vi "Create GCF LUT.vi"(8 "error in (no error)":errorcluster, 11 "C100L in":refnum<class "C100L.lvclass">) -> (0 "error out":errorcluster, 3 "C100L out":refnum<class "C100L.lvclass">)   [LabVIEW 2021, in "C100L.lvlib" / "C100L.lvclass"]
uses:
  C100L.lvclass
  GCF Data.ctl
  C100L.lvclass/C100L.ctl
  <vilib>/Utility/file.llb/Read Delimited Spreadsheet (string).vi
  <vilib>/BenjaminR/LookUp Table API/LUT.lvclass
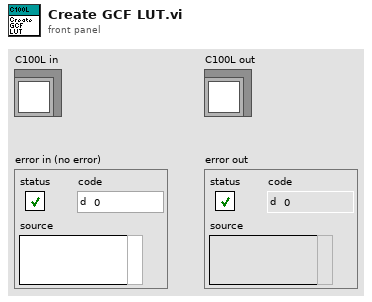
[diagram p1: front panel]
types:
  T1 = typedef "C100L.lvlib/C100L.lvclass/GCF Data.ctl" = map{string, dbl}
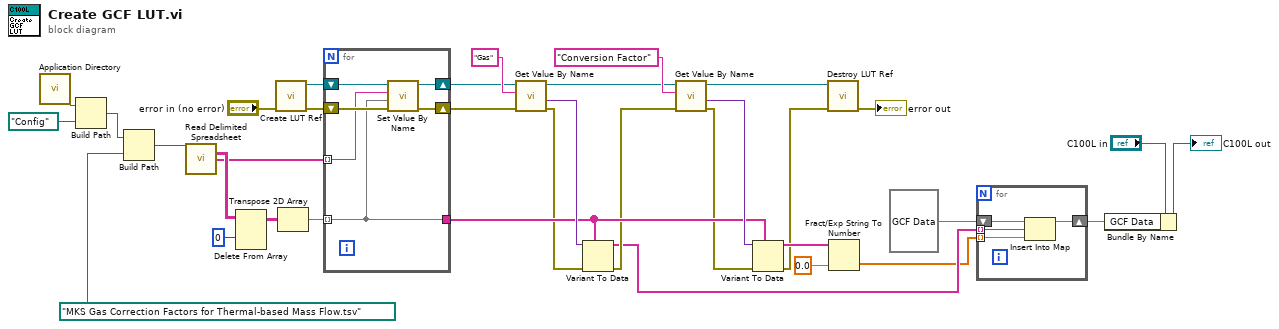
[diagram p0: block diagram]
diagram:
  n1 = call <vilib>:"Application Directory.vi"() -> ("Application Directory"=w5:path)
  n2 = Build Path(base path=w5, name or relative path=path "Config") -> (appended path=w3:path)
  n3 = Build Path(base path=w3, name or relative path=path "MKS Gas Correction Factors for Thermal-based Mass Flow.tsv" ("file path (dialog if empty)")) -> (appended path=w1:path)
  n4 = call-poly <vilib>:"Read Delimited Spreadsheet.vi"("file path (dialog if empty)"=w1) -> ("all rows"=w35:string[][], "first row"=w32:string[])  [unwired: 9 in, 4 out]
  n5 = Delete From Array(array=w35, index (row)=0) -> (array with subset deleted=w30:string[][])  [unwired: 2 in, 1 out]
  n6 = call <vilib>:"Create LUT Ref.vi"("error in (no error)"="error in (no error)") -> ("error out"=w31:errorcluster, "LUT out"=w33:refnum<class "LUT.lvclass">)  [unwired: 9 in]
  n7 = Transpose 2D Array(2D array=w30) -> (transposed array=w29:string[][])
  n8 = for {
    tunnel: w32 -> [w37] mode=indexing
    tunnel: w29 -> [w36] mode=indexing
    shift-right: [w40] -> w26
    shift-left: w33 -> [w41]
    shift-right: [w39] -> w27
    shift-left: w31 -> [w38]
    tunnel: [w36] -> w21
    n9 = call <vilib>:"Set Value By Name.vi"("error in (no error)"=w38, "Value"=w36, "Name"=w37, "LUT in"=w41) -> ("error out"=w39:errorcluster, "LUT out"=w40:refnum<class "LUT.lvclass">)  [unwired: 5 in, 1 out]
  }
  n10 = call <vilib>:"Get Value By Name.vi"("error in (no error)"=w27, "Name"="Gas", "LUT in"=w26) -> ("error out"=w15:errorcluster, "Value"=w25:variant, "LUT out"=w22:refnum<class "LUT.lvclass">)  [unwired: 5 in, 1 out]
  n11 = Variant To Data(error in=w15, type=w21, Variant=w25) -> (data=w9:string[], error out=w14:errorcluster)
  n12 = call <vilib>:"Get Value By Name.vi"("error in (no error)"=w14, "Name"="Conversion Factor", "LUT in"=w22) -> ("error out"=w13:errorcluster, "Value"=w24:variant, "LUT out"=w18:refnum<class "LUT.lvclass">)  [unwired: 5 in, 1 out]
  n13 = Variant To Data(error in=w13, type=w21, Variant=w24) -> (data=w20:string[], error out=w12:errorcluster)
  n14 = call <vilib>:"Destroy LUT Ref.vi"("error in (no error)"=w12, "LUT in"=w18) -> ("error out"=→"error out":errorcluster)  [unwired: 9 in]
  n15 = Fract/Exp String To Number(string=w20, default (0 dbl)=0.0 ("default (0 DBL)")) -> (number=w8:dbl[])  [unwired: 2 in, 1 out]
  n16 = for {
    tunnel: w9 -> [w45] mode=indexing
    tunnel: w8 -> [w44] mode=indexing
    shift-right: [w42] -> w11
    shift-left: T1 {} ("GCF Data") -> [w43]
    n17 = Insert Into Map(map in=w43, key=w45, value=w44) -> (map out=w42:T1)  [unwired: 2 out]
  }
  n18 = Bundle By Name(cluster="C100L in", "GCF Data"=w11) -> (→"C100L out":refnum<class "C100L.lvclass">)
